vi "arraypictring.vi"(1 "Array In":u16[](array[ring])) -> (0 "Array Out":u16[](array[ring]))   [LabVIEW 2012]
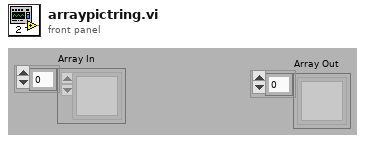
[diagram p1: front panel]
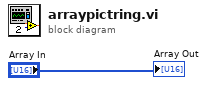
[diagram p0: block diagram]
diagram:
  "Array Out" <- "Array In"
